vi "Acquire Temperatures.vi"(8 "Error In":errorcluster, 11 "Settings in":T1) -> (0 "Error Out":errorcluster, 3 "Settings Out":T1)   [LabVIEW 2019, in "Acquisition.lvlib"]
uses:
  Acquisition.lvlib
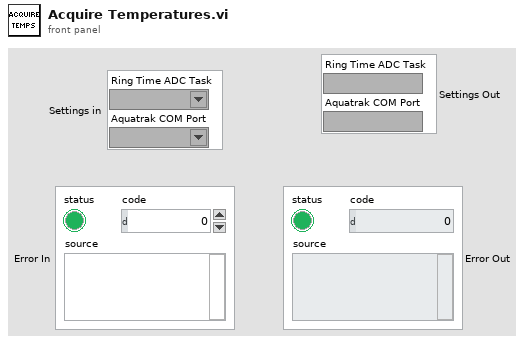
[diagram p1: front panel]
types:
  T1 = cluster{"Ring Time ADC Task":refnum<k21>, "Aquatrak COM Port":refnum<visa-resource-name>}
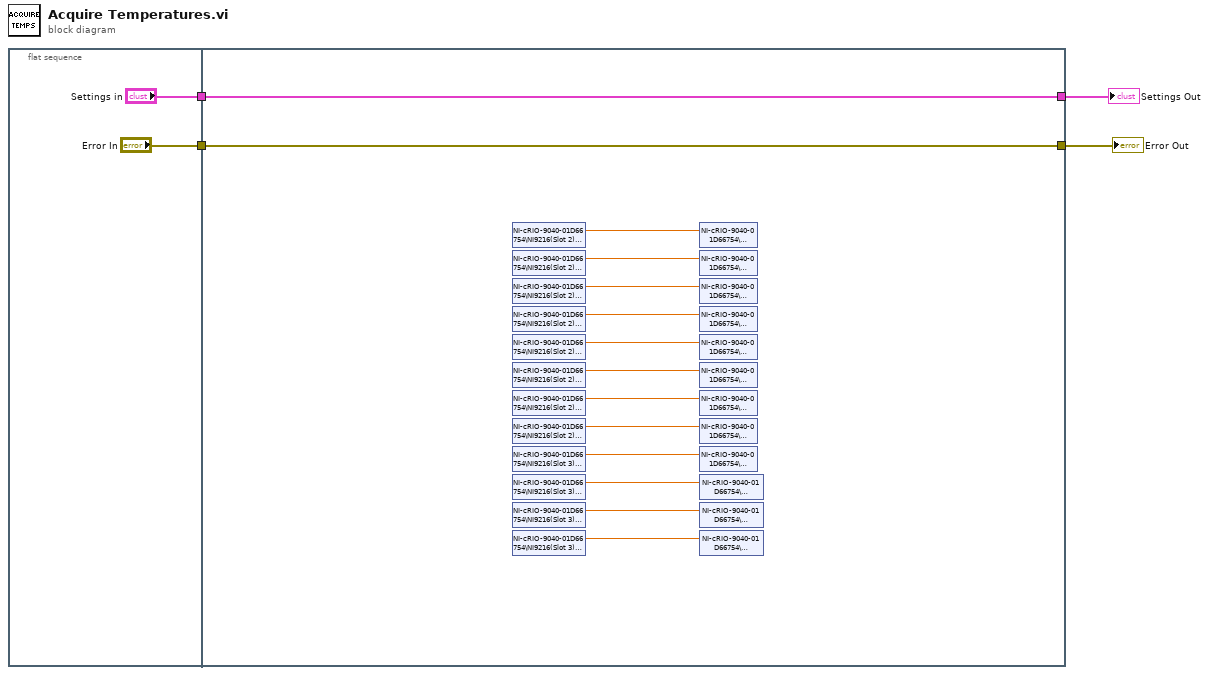
[diagram p0: block diagram]
diagram:
  n1 = flat-sequence {
    tunnel: ["Settings in"] -> w2
    tunnel: ["Error In"] -> w1
    tunnel: [w19] -> w3
    tunnel: [w20] -> w4
    tunnel: w2 -> [w20]
    tunnel: w1 -> [w19]
    frame #0 {
    }
    frame #1 {
      n2 = shared-variable "NI-cRIO-9040-01D66754\\NI9216(Slot 2)\\RTD0"() -> (w18:dbl)  [unwired: 1 in, 1 out]
      n3 = shared-variable "NI-cRIO-9040-01D66754\\NI9216(Slot 2)\\RTD1"() -> (w17:dbl)  [unwired: 1 in, 1 out]
      n4 = shared-variable "NI-cRIO-9040-01D66754\\NI9216(Slot 2)\\RTD2"() -> (w16:dbl)  [unwired: 1 in, 1 out]
      n5 = shared-variable "NI-cRIO-9040-01D66754\\NI9216(Slot 2)\\RTD3"() -> (w15:dbl)  [unwired: 1 in, 1 out]
      n6 = shared-variable "NI-cRIO-9040-01D66754\\NI9216(Slot 2)\\RTD4"() -> (w14:dbl)  [unwired: 1 in, 1 out]
      n7 = shared-variable "NI-cRIO-9040-01D66754\\NI9216(Slot 2)\\RTD5"() -> (w13:dbl)  [unwired: 1 in, 1 out]
      n8 = shared-variable "NI-cRIO-9040-01D66754\\NI9216(Slot 2)\\RTD6"() -> (w12:dbl)  [unwired: 1 in, 1 out]
      n9 = shared-variable "NI-cRIO-9040-01D66754\\NI9216(Slot 2)\\RTD7"() -> (w11:dbl)  [unwired: 1 in, 1 out]
      n10 = shared-variable "NI-cRIO-9040-01D66754\\NI9216(Slot 3)\\RTD0"() -> (w10:dbl)  [unwired: 1 in, 1 out]
      n11 = shared-variable "NI-cRIO-9040-01D66754\\NI9216(Slot 3)\\RTD1"() -> (w9:dbl)  [unwired: 1 in, 1 out]
      n12 = shared-variable "NI-cRIO-9040-01D66754\\NI9216(Slot 3)\\RTD2"() -> (w8:dbl)  [unwired: 1 in, 1 out]
      n13 = shared-variable "NI-cRIO-9040-01D66754\\NI9216(Slot 3)\\RTD3"() -> (w7:dbl)  [unwired: 1 in, 1 out]
      n14 = shared-variable "NI-cRIO-9040-01D66754\\NetworkVariables.lvlib\\T1"(w18) -> ()  [unwired: 1 in, 1 out]
      n15 = shared-variable "NI-cRIO-9040-01D66754\\NetworkVariables.lvlib\\T2"(w17) -> ()  [unwired: 1 in, 1 out]
      n16 = shared-variable "NI-cRIO-9040-01D66754\\NetworkVariables.lvlib\\T3"(w16) -> ()  [unwired: 1 in, 1 out]
      n17 = shared-variable "NI-cRIO-9040-01D66754\\NetworkVariables.lvlib\\T4"(w15) -> ()  [unwired: 1 in, 1 out]
      n18 = shared-variable "NI-cRIO-9040-01D66754\\NetworkVariables.lvlib\\T5"(w14) -> ()  [unwired: 1 in, 1 out]
      n19 = shared-variable "NI-cRIO-9040-01D66754\\NetworkVariables.lvlib\\T6"(w13) -> ()  [unwired: 1 in, 1 out]
      n20 = shared-variable "NI-cRIO-9040-01D66754\\NetworkVariables.lvlib\\T7"(w12) -> ()  [unwired: 1 in, 1 out]
      n21 = shared-variable "NI-cRIO-9040-01D66754\\NetworkVariables.lvlib\\T8"(w11) -> ()  [unwired: 1 in, 1 out]
      n22 = shared-variable "NI-cRIO-9040-01D66754\\NetworkVariables.lvlib\\T9"(w10) -> ()  [unwired: 1 in, 1 out]
      n23 = shared-variable "NI-cRIO-9040-01D66754\\NetworkVariables.lvlib\\T10"(w9) -> ()  [unwired: 1 in, 1 out]
      n24 = shared-variable "NI-cRIO-9040-01D66754\\NetworkVariables.lvlib\\T11"(w8) -> ()  [unwired: 1 in, 1 out]
      n25 = shared-variable "NI-cRIO-9040-01D66754\\NetworkVariables.lvlib\\T12"(w7) -> ()  [unwired: 1 in, 1 out]
    }
  }
  "Error Out" <- w3
  "Settings Out" <- w4
